vi "TEST-SAOMM-OffsetGUI.vi"(0 "Hexapod VRN":refnum<visa-resource-name>="COM4", 1 "Active Refnum":refnum<vi>, 2 "PrAMS-ACK":refnum<vi>, 7 "output cluster":T1, 13 "MessageType":cluster{string[], u32[]}={["emtError", "emtAreYouThere", "emtAcknowledgment", "emtGetClientType", "emtClientType", "emtGetImageExposureTime", "emtSetImageExposureTime", "emtImageExposureTime", "emtGetOptimalExposureTime", "emtSetOptimalExposureTime", "emtOptimalExposureTime", "emtGetImageEMGain", "emtSetImageEMGain", "emtImageEMGain", "emtGetFPGACtrl", "emtSetFPGACtrl", "emtFPGACtrl", "emtGetImageWidth", "emtSetImageWidth", "emtImageWidth", "emtGetImageHeight", "emtSetImageHeight", "emtImageHeight", "emtGetImageBinning", "emtSetImageBinning", "emtImageBinning", "emtGetImageDisplayFrameRate", "emtSetImageDisplayFrameRate", "emtImageDisplayFrameRate", "emtGetROIWidth", "emtSetROIWidth", "emtROIWidth", "emtGetROIHeight", "emtSetROIHeight", "emtROIHeight", "emtGetROIXOffset", "emtSetROIXOffset", "emtROIXOffset", "emtGetROIYOffset", "emtSetROIYOffset", "emtROIYOffset", "emtStartAcquisition", "mtStopAcquisition", "emtAcquisitionStarted", "emtAcquisitionStopped", "emtGetFalconImage", "emtFalconImage"], [1, 2, 3, 4, 5, 1001, 1101, 1201, 1002, 1102, 1202, 1003, 1103, 1203, 1004, 1104, 1204, 1005, 1105, 1205, 1006, 1106, 1206, 1007, 1107, 1207, 1008, 1108, 1208, 1009, 1109, 1209, 1010, 1110, 1210, 1011, 1111, 1211, 1012, 1112, 1212, 1130, 1131, 1150, 1151, 1070, 1270]}) -> (8 "Error":bool)   [LabVIEW 2019]
uses:
  Polymorphics/Num2littleEndian(DBL).vi
panel:
  out "First Run":bool
  in  "IncUV":dbl caption="Incrément" format="%.4g"
  in  "IncXYZ":dbl caption="Incrément" format="%.3f"
  in  "V+":bool
  in  "V-":bool
  in  "U+":bool
  in  "U-":bool
  in  "Z+":bool
  in  "Z-":bool
  in  "Y+":bool
  in  "Y-":bool
  in  "X+":bool
  in  "X-":bool
  in  "keep-active":bool caption="Laisser ouvert ?"
  in  "Signature":u32=1886544237
  in  "Cancel":bool
  in  "Send":bool
  in  "X":dbl caption="Pos" min=-5.0 max=5.0 format="%.4f"
  in  "Y":dbl caption="Pos" min=-5.0 max=5.0 format="%.4f"
  in  "Z":dbl caption="Pos" min=-5.0 max=5.0 format="%.4f"
  in  "U":dbl caption="Pos" min=-1.0 max=1.0 format="%.4f"
  in  "V":dbl caption="Pos" min=-1.0 max=1.0 format="%.4f"
  # "OFFSETS"
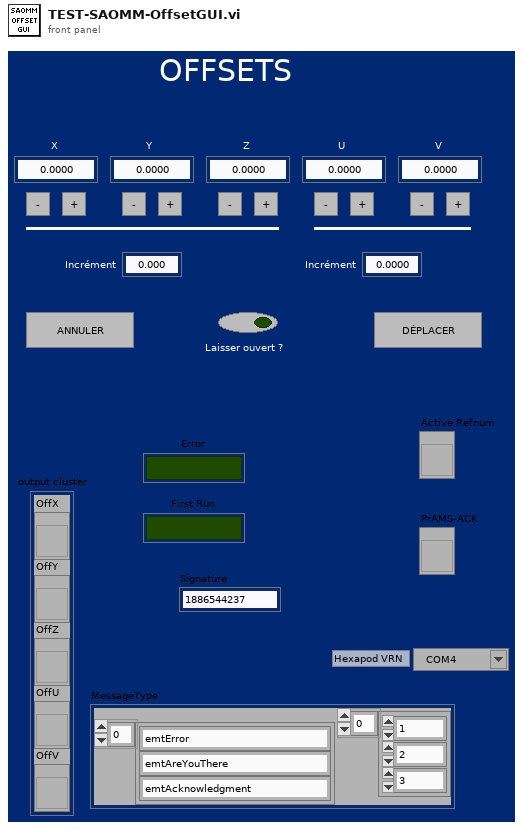
[diagram p1: front panel]
types:
  T1 = cluster{"OffX":refnum<vi>, "OffY":refnum<vi>, "OffZ":refnum<vi>, "OffU":refnum<vi>, "OffV":refnum<vi>}
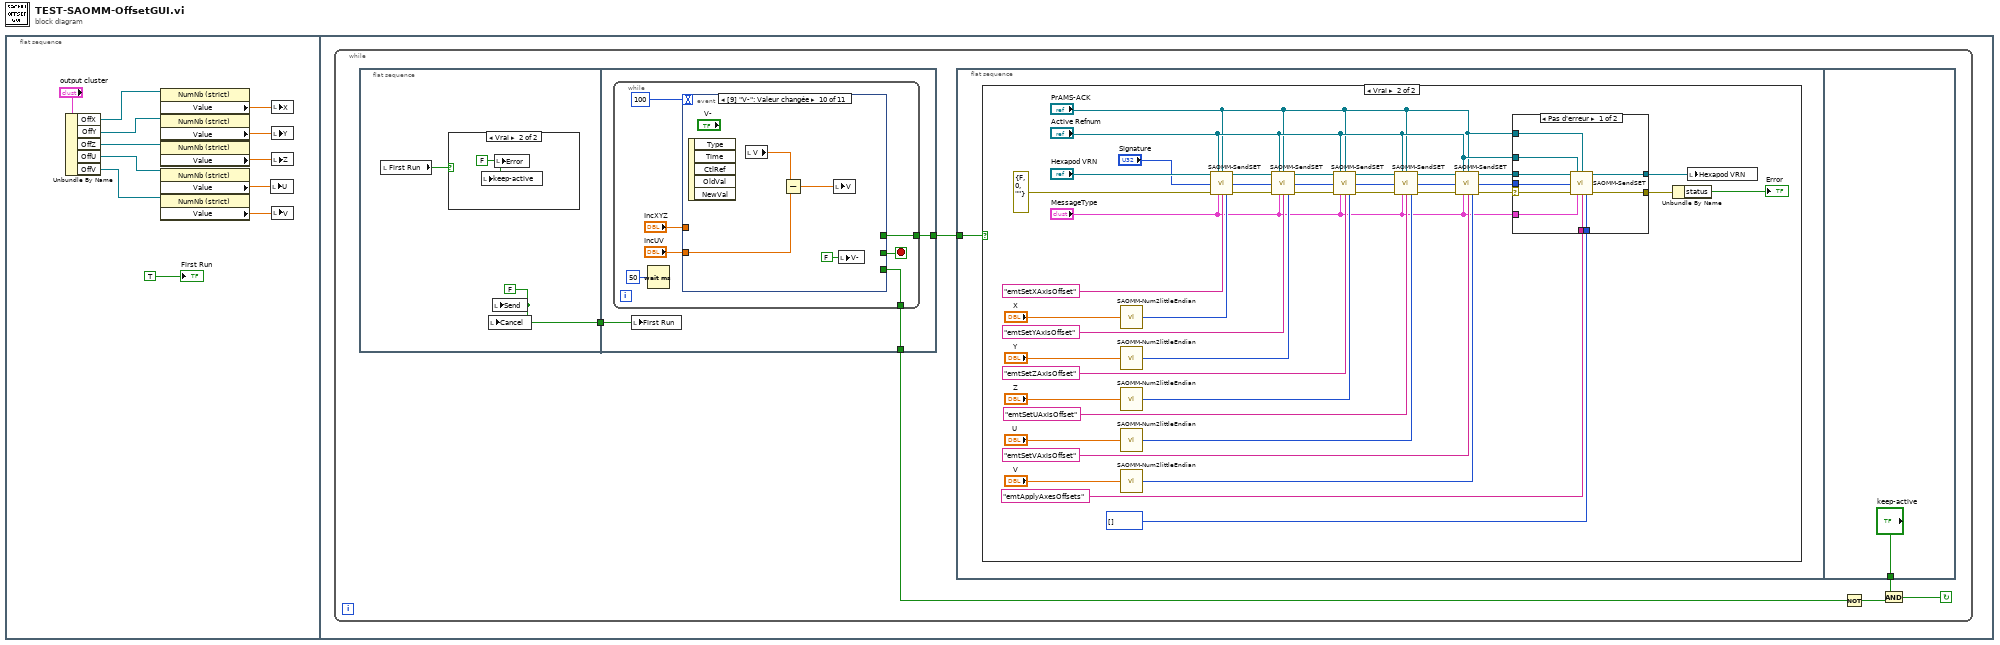
[diagram p0: block diagram]
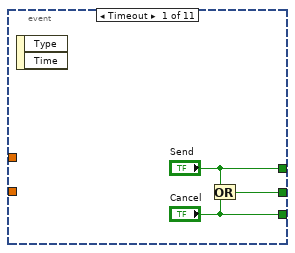
[diagram p5: hidden frame]
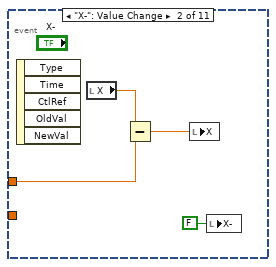
[diagram p6: hidden frame]
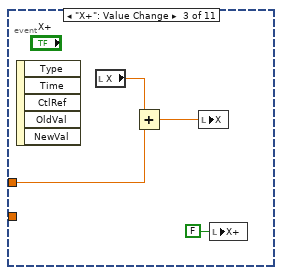
[diagram p7: hidden frame]
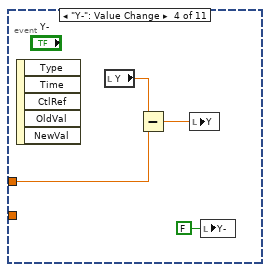
[diagram p8: hidden frame]
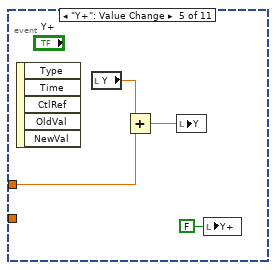
[diagram p9: hidden frame]
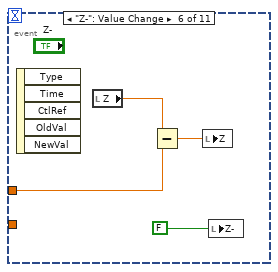
[diagram p10: hidden frame]
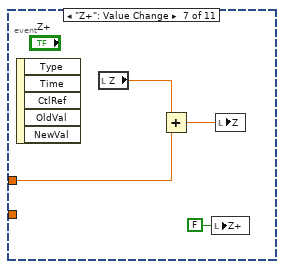
[diagram p11: hidden frame]
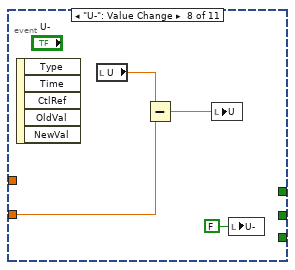
[diagram p12: hidden frame]
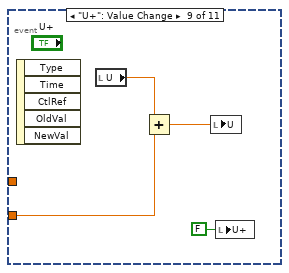
[diagram p13: hidden frame]
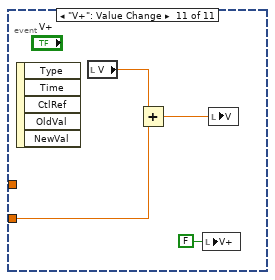
[diagram p14: hidden frame]
diagram:
  n1 = flat-sequence {
    frame #0 {
      n2 = Unbundle By Name("output cluster") -> ("OffX"=w10:refnum<vi>, "OffY"=w9:refnum<vi>, "OffZ"=w8:refnum<vi>, "OffU"=w7:refnum<vi>, "OffV"=w6:refnum<vi>)
      n3 = property class="NumNb (strict)"(reference=w10) -> ("Value"=w1:dbl)  [unwired: 1 in, 2 out]
      n4 = property class="NumNb (strict)"(reference=w9) -> ("Value"=w2:dbl)  [unwired: 1 in, 2 out]
      n5 = property class="NumNb (strict)"(reference=w8) -> ("Value"=w3:dbl)  [unwired: 1 in, 2 out]
      n6 = property class="NumNb (strict)"(reference=w7) -> ("Value"=w4:dbl)  [unwired: 1 in, 2 out]
      n7 = property class="NumNb (strict)"(reference=w6) -> ("Value"=w5:dbl)  [unwired: 1 in, 2 out]
      n8 = local write "U"(w4) -> ()
      n9 = local write "X"(w1) -> ()
      n10 = local write "Y"(w2) -> ()
      n11 = local write "Z"(w3) -> ()
      n12 = local write "V"(w5) -> ()
      "First Run" <- TRUE
    }
    frame #1 {
      n13 = while {
        stop <- w16 continue-if-true
        n14 = flat-sequence {
          tunnel: [w70] -> w13
          tunnel: [w73] -> w14
          tunnel: [w74] -> w18
          tunnel: w13 -> [w72]
          frame #0 {
            w70 = FALSE
            n15 = local read "First Run"() -> (w69:bool)
            n16 = case shown="Vrai" w69 {
              frame False {
              }
              frame True {
                w71 = FALSE ("Error")
                n17 = local write "keep-active"(w71) -> ()
                n18 = local write "Error"(w71) -> ()
              }
            }
            n19 = local write "Cancel"(w70) -> ()
            n20 = local write "Send"(w70) -> ()
          }
          frame #1 {
            n21 = while {
              tunnel: [w78] -> w74
              tunnel: [w77] -> w73
              stop <- w79 stop-if-true
              n22 = Wait (ms)(milliseconds to wait=u32 50) -> ()  [unwired: 1 out]
              n23 = event shown="[9] \"V-\": Valeur changée" {
                selector: _ -> [_ _ _ _ _ _ _ _ _ _ _]
                dyn-events: _ -> [_ _ _ _ _ _ _ _ _ _ _]
                timeout: 100 -> [_ _ _ _ _ _ _ _ _ _ _]
                tunnel: [w84 _ _ _ _ _ _ _ _ _ _] -> w79
                tunnel: ["Send" _ _ _ _ _ _ _ _ _ _] -> w78
                tunnel: ["Cancel" _ _ _ _ _ _ _ _ _ _] -> w77
                tunnel: "IncXYZ" -> [_ w88 w90 w94 w98 w104 w106 _ _ _ _]
                tunnel: "IncUV" -> [_ _ _ _ _ _ _ w110 w114 w119 w122]
                event Timeout {
                  n24 = event-data() -> ()  [unwired: 1 in, 2 out]
                  n25 = Or(x="Send", y="Cancel") -> (x .or. y?=w84:bool)
                }
                event "X-": Value Change {
                  n26 = event-data() -> ()  [unwired: 1 in, 5 out]
                  n27 = local read "X"() -> (w86:dbl)
                  n28 = Subtract(x=w86, y=w88) -> (x-y=w87:dbl)
                  n29 = local write "X"(w87) -> ()
                  n30 = local write "X-"(FALSE ("X-")) -> ()
                }
                event "X+": Value Change {
                  n31 = event-data() -> ()  [unwired: 1 in, 5 out]
                  n32 = local read "X"() -> (w91:dbl)
                  n33 = Add(x=w91, y=w90) -> (x+y=w92:dbl)
                  n34 = local write "X"(w92) -> ()
                  n35 = local write "X+"(FALSE ("X+")) -> ()
                }
                event "Y-": Value Change {
                  n36 = event-data() -> ()  [unwired: 1 in, 5 out]
                  n37 = local read "Y"() -> (w96:dbl)
                  n38 = Subtract(x=w96, y=w94) -> (x-y=w95:dbl)
                  n39 = local write "Y"(w95) -> ()
                  n40 = local write "Y-"(FALSE ("Y-")) -> ()
                }
                event "Y+": Value Change {
                  n41 = event-data() -> ()  [unwired: 1 in, 5 out]
                  n42 = local read "Y"() -> (w100:dbl)
                  n43 = Add(x=w100, y=w98) -> (x+y=w99:dbl)
                  n44 = local write "Y"(w99) -> ()
                  n45 = local write "Y+"(FALSE ("Y+")) -> ()
                }
                event "Z-": Value Change {
                  n46 = event-data() -> ()  [unwired: 1 in, 5 out]
                  n47 = local read "Z"() -> (w103:dbl)
                  n48 = Subtract(x=w103, y=w104) -> (x-y=w102:dbl)
                  n49 = local write "Z"(w102) -> ()
                  n50 = local write "Z-"(FALSE ("Z-")) -> ()
                }
                event "Z+": Value Change {
                  n51 = event-data() -> ()  [unwired: 1 in, 5 out]
                  n52 = local read "Z"() -> (w108:dbl)
                  n53 = Add(x=w108, y=w106) -> (x+y=w107:dbl)
                  n54 = local write "Z+"(FALSE ("Z+")) -> ()
                  n55 = local write "Z"(w107) -> ()
                }
                event "U-": Value Change {
                  n56 = event-data() -> ()  [unwired: 1 in, 5 out]
                  n57 = local read "U"() -> (w112:dbl)
                  n58 = Subtract(x=w112, y=w110) -> (x-y=w111:dbl)
                  n59 = local write "U"(w111) -> ()
                  n60 = local write "U-"(FALSE ("U-")) -> ()
                }
                event "U+": Value Change {
                  n61 = event-data() -> ()  [unwired: 1 in, 5 out]
                  n62 = local read "U"() -> (w116:dbl)
                  n63 = Add(x=w116, y=w114) -> (x+y=w115:dbl)
                  n64 = local write "U"(w115) -> ()
                  n65 = local write "U+"(FALSE ("U+")) -> ()
                }
                event "V-": Value Change {
                  n66 = event-data() -> ()  [unwired: 1 in, 5 out]
                  n67 = local read "V"() -> (w120:dbl)
                  n68 = Subtract(x=w120, y=w119) -> (x-y=w118:dbl)
                  n69 = local write "V"(w118) -> ()
                  n70 = local write "V-"(FALSE ("V-")) -> ()
                }
                event "V+": Value Change {
                  n71 = event-data() -> ()  [unwired: 1 in, 5 out]
                  n72 = local read "V"() -> (w124:dbl)
                  n73 = Add(x=w124, y=w122) -> (x+y=w123:dbl)
                  n74 = local write "V+"(FALSE ("V+")) -> ()
                  n75 = local write "V"(w123) -> ()
                }
              }
            }
            n76 = local write "First Run"(w72) -> ()
          }
        }
        n77 = flat-sequence {
          tunnel: w18 -> [w19]
          tunnel: ["keep-active"] -> w17
          frame #0 {
            n78 = case shown="Vrai" w19 {
              frame False {
              }
              frame True {
                n79 = call-poly "SAOMM-Num2littleEndian.vi"("Number"="X") -> ("LiitleEndianedData"=w42:u8[])  [unwired: 14 in]
                n80 = call-poly "SAOMM-Num2littleEndian.vi"("Number"="Y") -> ("LiitleEndianedData"=w43:u8[])  [unwired: 14 in]
                n81 = call-poly "SAOMM-Num2littleEndian.vi"("Number"="Z") -> ("LiitleEndianedData"=w44:u8[])  [unwired: 14 in]
                n82 = call-poly "SAOMM-Num2littleEndian.vi"("Number"="U") -> ("LiitleEndianedData"=w47:u8[])  [unwired: 14 in]
                n83 = call-poly "SAOMM-Num2littleEndian.vi"("Number"="V") -> ("LiitleEndianedData"=w48:u8[])  [unwired: 14 in]
                n84 = call "SAOMM-SendSET.vi"("PRAMMS-COMM IN"="Hexapod VRN", "Active Refnum"="Active Refnum", "PrAMS-ACK"="PrAMS-ACK", "Signature"="Signature", "Error IN"=errorcluster {"status"=FALSE, "code"=0, "source"=""}, "MessageType"="MessageType", "Active SET"="emtSetXAxisOffset", "Value (little endianed byte array)"=w42) -> ("PRAMMS-COMM OUT"=w33:refnum<visa-resource-name>, "Error OUT"=w39:errorcluster)  [unwired: 4 in, 2 out]
                n85 = call "SAOMM-SendSET.vi"("PRAMMS-COMM IN"=w33, "Active Refnum"="Active Refnum", "PrAMS-ACK"="PrAMS-ACK", "Signature"="Signature", "Error IN"=w39, "MessageType"="MessageType", "Active SET"="emtSetYAxisOffset", "Value (little endianed byte array)"=w43) -> ("PRAMMS-COMM OUT"=w34:refnum<visa-resource-name>, "Error OUT"=w38:errorcluster)  [unwired: 4 in, 2 out]
                n86 = call "SAOMM-SendSET.vi"("PRAMMS-COMM IN"=w34, "Active Refnum"="Active Refnum", "PrAMS-ACK"="PrAMS-ACK", "Signature"="Signature", "Error IN"=w38, "MessageType"="MessageType", "Active SET"="emtSetZAxisOffset", "Value (little endianed byte array)"=w44) -> ("PRAMMS-COMM OUT"=w54:refnum<visa-resource-name>, "Error OUT"=w37:errorcluster)  [unwired: 4 in, 2 out]
                n87 = call "SAOMM-SendSET.vi"("PRAMMS-COMM IN"=w54, "Active Refnum"="Active Refnum", "PrAMS-ACK"="PrAMS-ACK", "Signature"="Signature", "Error IN"=w37, "MessageType"="MessageType", "Active SET"="emtSetUAxisOffset", "Value (little endianed byte array)"=w47) -> ("PRAMMS-COMM OUT"=w55:refnum<visa-resource-name>, "Error OUT"=w36:errorcluster)  [unwired: 4 in, 2 out]
                n88 = call "SAOMM-SendSET.vi"("PRAMMS-COMM IN"=w55, "Active Refnum"="Active Refnum", "PrAMS-ACK"="PrAMS-ACK", "Signature"="Signature", "Error IN"=w36, "MessageType"="MessageType", "Active SET"="emtSetVAxisOffset", "Value (little endianed byte array)"=w48) -> ("PRAMMS-COMM OUT"=w53:refnum<visa-resource-name>, "Error OUT"=w52:errorcluster)  [unwired: 4 in, 2 out]
                n89 = case shown="Pas d'erreur" w52 {
                  selector: w52 -> [w57 w66]
                  tunnel: "Active Refnum" -> [w65 _]
                  tunnel: "PrAMS-ACK" -> [w64 _]
                  tunnel: "Signature" -> [w63 _]
                  tunnel: [w62 w67] -> w35
                  tunnel: [w61 w66] -> w21
                  tunnel: "MessageType" -> [w60 _]
                  tunnel: "emtApplyAxesOffsets" -> [w59 _]
                  tunnel: u8[] [] ("Value (little endianed byte array)") -> [w58 _]
                  tunnel: w53 -> [w56 w67]
                  frame No Error {
                    n90 = call "SAOMM-SendSET.vi"("PRAMMS-COMM IN"=w56, "Active Refnum"=w65, "PrAMS-ACK"=w64, "Signature"=w63, "Error IN"=w57, "MessageType"=w60, "Active SET"=w59, "Value (little endianed byte array)"=w58) -> ("PRAMMS-COMM OUT"=w62:refnum<visa-resource-name>, "Error OUT"=w61:errorcluster)  [unwired: 4 in, 2 out]
                  }
                  frame Error {
                  }
                }
                n91 = Unbundle By Name(w21) -> ("status"=→"Error":bool)
                n92 = local write "Hexapod VRN"(w35) -> ()
              }
            }
          }
          frame #1 {
          }
        }
        n93 = Not(x=w14) -> (.not. x?=w15:bool)
        n94 = And(x=w17, y=w15) -> (x .and. y?=w16:bool)
      }
    }
  }
